vi "Get Kasli Name from Alias.vi"(8 "error in (no error)":errorcluster, 10 "Kasli Alias":string, 11 "Kasli in":refnum<class "Kasli.lvclass">) -> (0 "error out":errorcluster, 2 "Kasli Name":string, 3 "Kasli out":refnum<class "Kasli.lvclass">)   [LabVIEW 2020, in "Kasli Wrapper 2.0.lvlib" / "Kasli.lvclass"]
uses:
  Kasli.lvclass
  Kasli.lvclass/Kasli.ctl
  f74609e2-d7b5-4696-a2f7-77896b9945e1.vi
  f74609e2-d7b5-4696-a2f7-77896b9945e1.vi/d4db2432-cc9c-482c-8957-dac855435ef6.vi
  f74609e2-d7b5-4696-a2f7-77896b9945e1.vi/86fbf154-bd7b-49a2-8ab2-a837b2a95f24.vi
  f74609e2-d7b5-4696-a2f7-77896b9945e1.vi/3b95b01e-1ec2-4565-bcd9-7606a5281010.vi
  f74609e2-d7b5-4696-a2f7-77896b9945e1.vi/96a08935-737a-44b2-979c-a81d56408f7e.vi
  f74609e2-d7b5-4696-a2f7-77896b9945e1.vi/d4db2432-cc9c-482c-8957-dac855435ef6.vi/6eaecd13-6e48-4772-a921-b51ebdf84d88.vi
  f74609e2-d7b5-4696-a2f7-77896b9945e1.vi/d4db2432-cc9c-482c-8957-dac855435ef6.vi/d2d5f2b7-06f4-47f6-971c-049c3fdbb653.vi
  f74609e2-d7b5-4696-a2f7-77896b9945e1.vi/3b95b01e-1ec2-4565-bcd9-7606a5281010.vi/6eaecd13-6e48-4772-a921-b51ebdf84d88.vi
  f74609e2-d7b5-4696-a2f7-77896b9945e1.vi/3b95b01e-1ec2-4565-bcd9-7606a5281010.vi/d2d5f2b7-06f4-47f6-971c-049c3fdbb653.vi
  f74609e2-d7b5-4696-a2f7-77896b9945e1.vi/96a08935-737a-44b2-979c-a81d56408f7e.vi/6eaecd13-6e48-4772-a921-b51ebdf84d88.vi
  f74609e2-d7b5-4696-a2f7-77896b9945e1.vi/96a08935-737a-44b2-979c-a81d56408f7e.vi/d2d5f2b7-06f4-47f6-971c-049c3fdbb653.vi
  <vilib>/Comparison/Less/Less Functor/Less Functor.lvclass
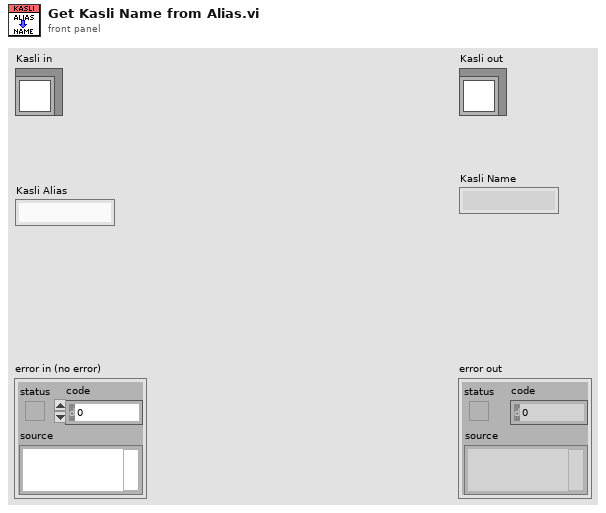
[diagram p1: front panel]
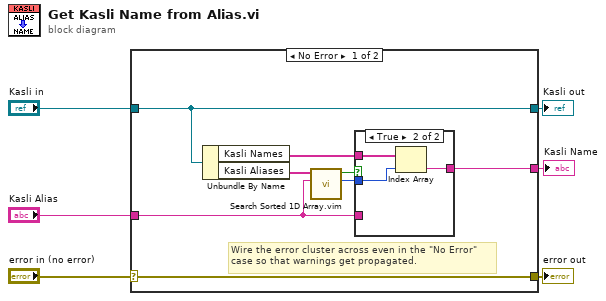
[diagram p0: block diagram]
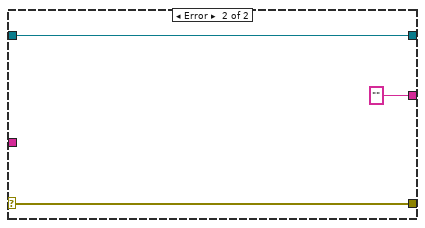
[diagram p3: hidden frame]
diagram:
  n1 = case shown="No Error" "error in (no error)" {
    selector: "error in (no error)" -> [w14 w21]
    tunnel: [w14 w21] -> w5
    tunnel: [w13 w20] -> w3
    tunnel: "Kasli in" -> [w13 w20]
    tunnel: "Kasli Alias" -> [w7 _]
    tunnel: [w9 "" ("IP")] -> w1
    frame No Error {
      # "Wire the error cluster across even in the \"No Error\"\ncase so that warnings get propagated."
      n2 = Unbundle By Name(w13) -> ("Kasli Names"=w11:string[], "Kasli Aliases"=w12:string[])
      n3 = call "Search Sorted 1D Array.vim"("element"=w7, "sorted 1D array"=w12) -> ("nearest index"=w10:i32, "found?"=w8:bool)  [unwired: 8 in]
      n4 = case shown="True" w8 {
        tunnel: w11 -> [_ w18]
        tunnel: w10 -> [_ w17]
        tunnel: [w15 w16] -> w9
        tunnel: w7 -> [w15 _]
        frame False {
        }
        frame True {
          n5 = Index Array(array=w18, index=w17) -> (element=w16:string)
        }
      }
    }
    frame Error {
    }
  }
  "error out" <- w5
  "Kasli out" <- w3
  "Kasli Name" <- w1
